vi "数据转换子程序.vi"(1 "formular in[0]":T2) -> (0 "output cluster":T1)   [LabVIEW 2021]
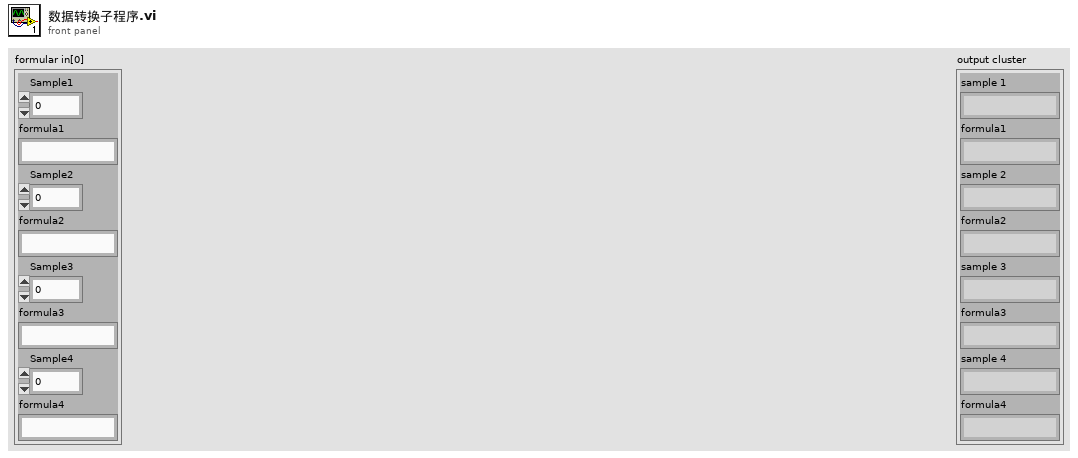
[diagram p1: front panel]
types:
  T1 = cluster{"sample 1":string, "formula1":string, "sample 2":string, "formula2":string, "sample 3":string, "formula3":string, "sample 4":string, "formula4":string}
  T2 = cluster{"Sample1":dbl, "formula1":string, "Sample2":dbl, "formula2":string, "Sample3":dbl, "formula3":string, "Sample4":dbl, "formula4":string}
  T3 = cluster{"formula1":string, "formula1":string, "formula1":string, "formula2":string, "formula1":string, "formula3":string, "formula1":string, "formula4":string}
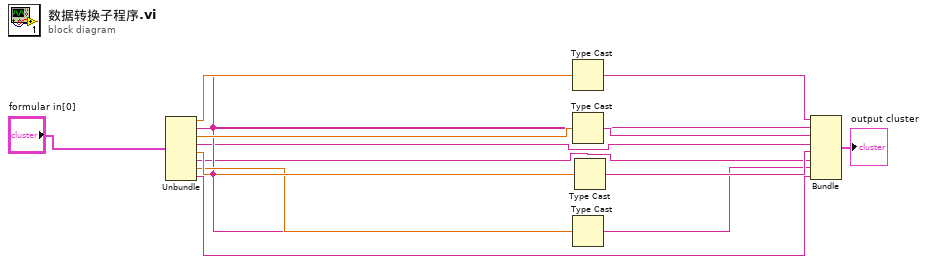
[diagram p0: block diagram]
diagram:
  n1 = Unbundle("formular in[0]") -> ("Sample1"=w13:dbl, "formula1"=w7:string, "Sample2"=w12:dbl, "formula2"=w6:string, "Sample3"=w11:dbl, "formula3"=w4:string, "Sample4"=w10:dbl, "formula4"=w2:string)
  n2 = Type Cast(type=w7, x=w13) -> (*(type *) &x=w9:string)
  n3 = Type Cast(type=w7, x=w12) -> (*(type *) &x=w8:string)
  n4 = Type Cast(type=w7, x=w10) -> (*(type *) &x=w3:string)
  n5 = Type Cast(type=w7, x=w11) -> (*(type *) &x=w5:string)
  n6 = Bundle("formula1"=w9, "formula1"=w7, "formula1"=w8, "formula2"=w6, "formula1"=w5, "formula3"=w4, "formula1"=w3, "formula4"=w2) -> (→"output cluster":T3)  [unwired: 1 in]
